vi "oa_Get the Index of the 1st Point in One Cycle (1 Channel).vi"(0 "resampled signal":cluster{"r0":dbl, "dr":dbl, "Y":dbl[]}={"r0"=0.0, "dr"=1.0, "Y"=[]} {"r0" format="%.2p"; "dr" format="%.2p"; "Y" format="%.2f"}, 1 "reset? (True)":bool=TRUE, 7 "speed profile":T1 {"speed [RPM]" format="%.2f"; "time [s]" format="%.2f"}, 9 "interpolated pulse positions":dbl[](array[numeric]) format="%.2f", 11 "error in (no error)":errorcluster, 12 "index mode":u16(ring) items=["round to nearest", "round to ceiling"]) -> (4 "resampled signal out":cluster{"r0":dbl, "dr":dbl, "Y":dbl[]}={"r0"=0.0, "dr"=1.0, "Y"=[]} {"r0" format="%.2p"; "dr" format="%.2p"; "Y" format="%.2f"}, 10 "interpolated pulse positions out":dbl[](array[numeric]), 15 "error out":errorcluster)   [LabVIEW 2017, in "SoundVib_Resampling.lvlib"]
uses:
  <vilib>/addons/Sound and Vibration/Order Analysis/Resample Order Tracking/SoundVib_Resampling.lvlib
  <vilib>/addons/Sound and Vibration/Order Analysis/Tach Process/SubVIs/speed profile.ctl
  <vilib>/addons/Sound and Vibration/Order Analysis/Tach Process/SoundVib_TachProcess.lvlib
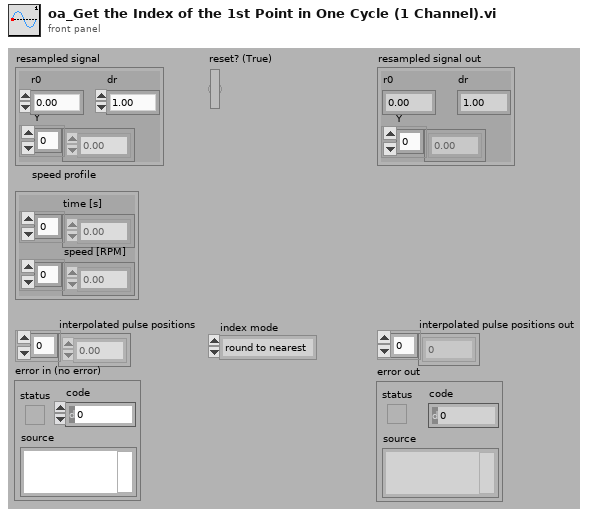
[diagram p1: front panel]
types:
  T1 = typedef "SoundVib_TachProcess.lvlib/speed profile.ctl" = cluster{"time [s]":dbl[], "speed [RPM]":dbl[]}
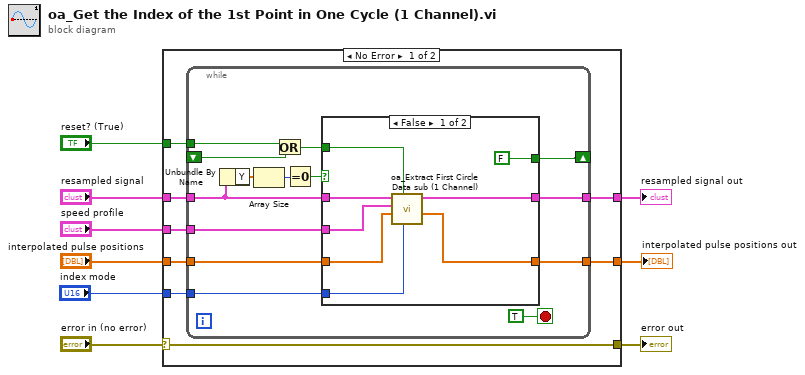
[diagram p0: block diagram]
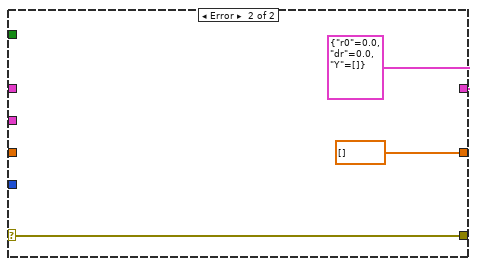
[diagram p3: hidden frame]
diagram:
  n1 = case shown="No Error" "error in (no error)" {
    selector: "error in (no error)" -> [w12 w45]
    tunnel: [w12 w45] -> w8
    tunnel: "reset? (True)" -> [w17 _]
    tunnel: "resampled signal" -> [w16 _]
    tunnel: [w15 cluster{"r0":dbl, "dr":dbl, "Y":dbl[]} {"r0"=0.0, "dr"=0.0, "Y"=[]} ("resampled signal")] -> w5
    tunnel: "speed profile" -> [w14 _]
    tunnel: "interpolated pulse positions" -> [w13 _]
    tunnel: [w11 dbl[] []] -> w2
    tunnel: "index mode" -> [w10 _]
    frame No Error {
      n2 = while {
        tunnel: w17 -> [w24]
        tunnel: w16 -> [w27]
        tunnel: [w31] -> w15
        tunnel: w14 -> [w30]
        tunnel: w13 -> [w29]
        shift-right: [w23] -> _
        shift-left: _ -> [w20]
        tunnel: [w19] -> w11
        tunnel: w10 -> [w18]
        stop <- TRUE stop-if-true
        n3 = Unbundle By Name(w27) -> ("Y"=w26:dbl[])
        n4 = Array Size(array=w26) -> (size(s)=w25:i32)
        n5 = Or(x=w24, y=w20) -> (x .or. y?=w21:bool)
        n6 = Equal To 0?(x=w25) -> (x = 0?=w22:bool)
        n7 = case shown="False" w22 {
          tunnel: [w39 w41] -> w31
          tunnel: w30 -> [w38 _]
          tunnel: w29 -> [w37 w40]
          tunnel: w27 -> [w36 w41]
          tunnel: [FALSE w42] -> w23
          tunnel: w21 -> [w34 w42]
          tunnel: [w33 w40] -> w19
          tunnel: w18 -> [w32 _]
          frame False {
            n8 = call <vilib>:"oa_Extract First Circle Data sub (1 Channel).vi"("index mode"=w32, "reset? (True)"=w34, "interpolated pulse positions"=w37, "speed profile"=w38, "resampled signal"=w36) -> ("interpolated pulse positions out"=w33:dbl[], "resampled signal out"=w39:cluster{"r0":dbl, "dr":dbl, "Y":dbl[]})  [unwired: 5 in]
          }
          frame True {
          }
        }
      }
    }
    frame Error {
    }
  }
  "error out" <- w8
  "resampled signal out" <- w5
  "interpolated pulse positions out" <- w2
